vi "Set Camera Light Intensity.vi"(8 "error in (no error)":errorcluster, 9 "camera name":string, 10 "Intensity":dbl, 11 "Gantry Class in":refnum<class "Gantry.lvclass">) -> (0 "error out":errorcluster, 3 "Gantry Class out":refnum<class "Gantry.lvclass">)   [LabVIEW 2026, in "Gantry.lvclass"]
uses:
  Gantry.lvclass
  <instrlib>/Aerotech Automation1/Commands/IO/typedefs/AnalogOutputSet parameters.ctl
  <vilib>/DAQmx/write.llb/DAQmx Write (Analog DBL 1Chan 1Samp).vi
  <vilib>/DAQmx/create/channels.llb/DAQmx Create Channel (AO-Voltage-Basic).vi
  <vilib>/DAQmx/miscellaneous.llb/DAQmx Fill In Error Info.vi
  Gantry.lvclass/Gantry.ctl
  FlexWorktable/FlexWorktable.lvclass
  <instrlib>/Aerotech Automation1/Aerotech Automation1.lvlib
  GH2/GH2.lvclass
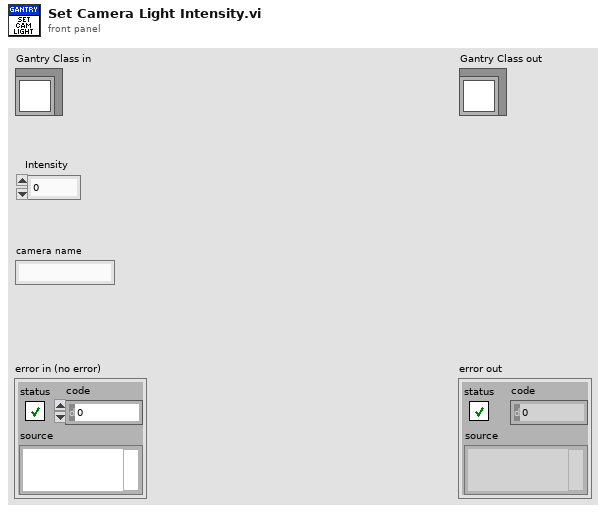
[diagram p1: front panel]
types:
  T1 = typedef "Aerotech Automation1.lvlib/AnalogOutputSet parameters.ctl" = cluster{"value":dbl, "outputNum":i64, "axis":string}
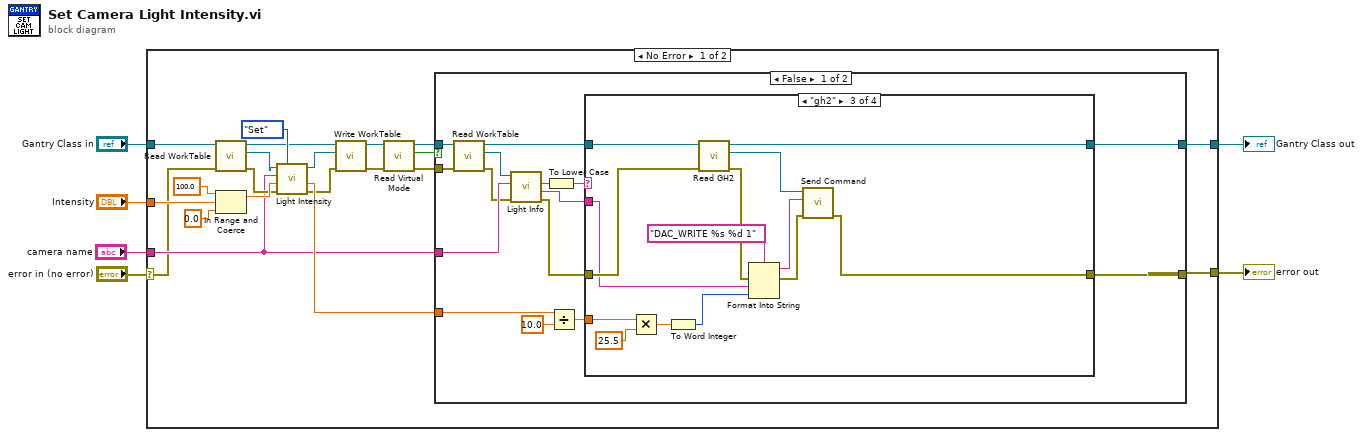
[diagram p0: block diagram]
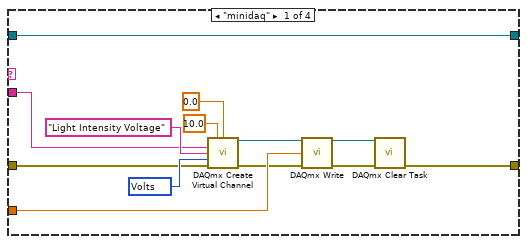
[diagram p2: hidden frame]
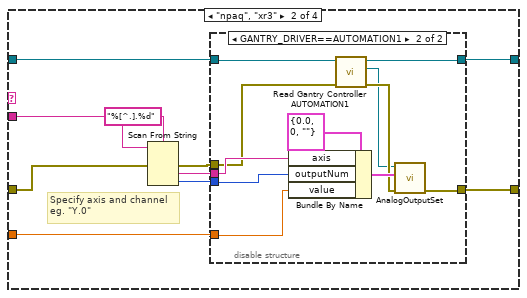
[diagram p3: hidden frame]
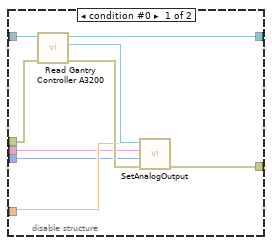
[diagram p4: hidden frame]
diagram:
  n1 = case shown="No Error" "error in (no error)" {
    selector: "error in (no error)" -> [w9 w105]
    tunnel: [w24 w105] -> w5
    tunnel: [w25 w104] -> w3
    tunnel: "Gantry Class in" -> [w15 w104]
    tunnel: "Intensity" -> [w11 _]
    tunnel: "camera name" -> [w16 _]
    frame No Error {
      n2 = call-dynamic "Read WorkTable.vi"("error in"=w9, "Gantry Class in"=w15) -> ("error out"=w18:errorcluster, "Worktable"=w21:refnum<class "FlexWorktable.lvclass">, "Gantry Class out"=w14:refnum<class "Gantry.lvclass">)  [unwired: 7 in]
      n3 = In Range and Coerce(upper limit=100.0, x=w11, lower limit=0.0) -> (coerced(x)=w19:dbl)  [unwired: 1 out]
      n4 = call "Light Intensity.vi"("Get/Set"=enum16{"Get", "Set"}."Set", "error in (no error)"=w18, "Intensity In"=w19, "Light Name"=w16, "FlexWorktable in"=w21) -> ("error out"=w12:errorcluster, "Intensity out"=w17:dbl, "FlexWorktable out"=w13:refnum<class "FlexWorktable.lvclass">)  [unwired: 4 in]
      n5 = call-dynamic "Write WorkTable.vi"("error in (no error)"=w12, "FlexWorktable"=w13, "Gantry Class in"=w14) -> ("error out"=w8:errorcluster, "Gantry Class out"=w10:refnum<class "Gantry.lvclass">)  [unwired: 7 in]
      n6 = call-dynamic "Read Virtual Mode.vi"("error in (no error)"=w8, "Gantry in"=w10) -> ("error out"=w7:errorcluster, "Is Virtual"=w27:bool, "Gantry out"=w26:refnum<class "Gantry.lvclass">)  [unwired: 6 in, 1 out]
      n7 = case shown="False" w27 {
        tunnel: w26 -> [w37 w103]
        tunnel: [w42 w103] -> w25
        tunnel: w7 -> [w32 w102]
        tunnel: [w41 w102] -> w24
        tunnel: w17 -> [w34 _]
        tunnel: w16 -> [w33 _]
        frame False {
          n8 = call-dynamic "Read WorkTable.vi"("error in"=w32, "Gantry Class in"=w37) -> ("error out"=w31:errorcluster, "Worktable"=w36:refnum<class "FlexWorktable.lvclass">, "Gantry Class out"=w35:refnum<class "Gantry.lvclass">)  [unwired: 7 in]
          n9 = call "Light Info.vi"("error in (no error)"=w31, "Light Name"=w33, "FlexWorktable in"=w36) -> ("error out"=w30:errorcluster, "hardware_address"=w38:string, "control"=w29:string)  [unwired: 5 in, 1 out]
          n10 = To Lower Case(string=w29) -> (all lower case string=w28:string)
          n11 = Divide(x=w34, y=10.0) -> (x/y=w39:dbl)
          n12 = case shown="\"gh2\"" w28 {
            tunnel: w35 -> [w55 w63 w98 w101]
            tunnel: w30 -> [w48 w62 w97 w100]
            tunnel: [w55 w58 w99 w101] -> w42
            tunnel: [w43 w57 w86 w100] -> w41
            tunnel: w39 -> [w54 w61 w95 _]
            tunnel: w38 -> [w46 w65 w90 _]
            frame "minidaq" {
              w52 = 10348 items=["Volts"=10348, "From Custom Scale"=10065] ("units")
              n13 = call-poly <vilib>:"DAQmx Create Virtual Channel.vi"("maximum value"=10.0, "minimum value"=0.0, "physical channels"=w46, "name to assign"="Light Intensity Voltage", "units"=w52, "error in"=w48) -> ("task out"=w49:refnum<k21>, "error out"=w47:errorcluster)  [unwired: 8 in]
              n14 = call-poly <vilib>:"DAQmx Write.vi"("task/channels in"=w49, "data"=w54, "error in"=w47) -> ("task out"=w45:refnum<k21>, "error out"=w44:errorcluster)  [unwired: 10 in, 1 out]
              n15 = call <vilib>:"DAQmx Clear Task.vi"("task in"=w45, "error in"=w44) -> ("error out"=w43:errorcluster)  [unwired: 13 in]
            }
            frame "npaq", "xr3" {
              # "Specify axis and channel\neg. \"Y.0\""
              n16 = Scan From String(format string="%[^.].%d", input string=w65, error in=w62) -> (error out=w56:errorcluster, output 1=w59:string, output 2=w60:i32)  [unwired: 3 in, 2 out]
              n17 = disable-structure shown="GANTRY_DRIVER==AUTOMATION1" {
                disable-tunnel: w63 -> [w72 w77]
                disable-tunnel: w61 -> [w69 w81]
                disable-tunnel: w60 -> [w68 w80]
                disable-tunnel: w59 -> [w67 w79]
                disable-tunnel: [w71 w76] -> w58
                disable-tunnel: [w70 w75] -> w57
                disable-tunnel: w56 -> [w66 w78]
                frame condition #0 {
                  n18 = call "Read Gantry Controller A3200.vi"("error in (no error)"=w66, "Gantry in"=w72) -> ("error out"=w74:errorcluster, "A3200 controller out"=w73:refnum<k24>, "Gantry out"=w71:refnum<class "Gantry.lvclass">)  [unwired: 7 in]
                  n19 = call "SetAnalogOutput.vi"("value"=w69, "channel"=w68, "error in (no error)"=w74, "axis name"=w67, "controller in"=w73) -> ("error out"=w70:errorcluster)  [unwired: 5 in, 1 out]
                }
                frame condition #1 (active) {
                  n20 = Bundle By Name(cluster=T1 {"value"=0.0, "outputNum"=0, "axis"=""} ("AnalogOutputSet parameters"), "axis"=w79, "outputNum"=w80, "value"=w81) -> (w85:T1)
                  n21 = call "Read Gantry Controller AUTOMATION1.vi"("error in (no error)"=w78, "Gantry in"=w77) -> ("error out"=w83:errorcluster, "Controller AUTOMATION1"=w82:refnum<k24>, "Gantry out"=w76:refnum<class "Gantry.lvclass">)  [unwired: 7 in]
                  n22 = call <instrlib>:"AnalogOutputSet.vi"("error in (no error)"=w83, "AnalogOutputSet parameters"=w85, "Controller Refnum"=w82) -> ("error out"=w75:errorcluster)  [unwired: 7 in, 1 out]
                }
              }
            }
            frame "gh2" {
              n23 = Multiply(x=w95, y=25.5) -> (x*y=w93:dbl)
              n24 = To Word Integer(number=w93) -> (16bit integer=w91:i16)
              n25 = call "Read GH2.vi"("error in (no error)"=w97, "Gantry in"=w98) -> ("error out"=w88:errorcluster, "GH2.lvclass"=w92:refnum<class "GH2.lvclass">, "Gantry out"=w99:refnum<class "Gantry.lvclass">)  [unwired: 7 in]
              n26 = Format Into String(format string="DAC_WRITE %s %d 1", error in=w88, w90, w91) -> (resulting string=w89:string, error out=w87:errorcluster)  [unwired: 1 in]
              n27 = call "Send Command.vi"("error in (no error)"=w87, "command"=w89, "GH2 in"=w92) -> ("error out"=w86:errorcluster)  [unwired: 6 in, 2 out]
            }
            frame "manual", Default {
              # "control is manual, do nothing here."
            }
          }
        }
        frame True {
          # "Virtual Mode: Do nothing"
        }
      }
    }
    frame Error {
    }
  }
  "error out" <- w5
  "Gantry Class out" <- w3
